vi "CreateExperimentRunsNode.vi"(8 "Error In":errorcluster, 10 "Experiment":T1={"File Path"=path "", "Operator"="Operator", "Project"="Project Description", "Target Dose (dpa)"=0.0, "Sample"={"Name"="", "Description"="", "Molar Mass (g/mol)"=0.0, "Density (g/cm^3)"=0.0, "Irradiation Area (cm^2)"=0.0, "SRIM Damage Peak (disp * ions/cm)"=0.0}, "Beam Line"={"Type"=enum."Ion Beam Analysis", "Ion"=enum."H", "Charge State"=0, "Total Source Ion Energy (kV)"=nan}, "Runs"=[]} {"Beam Line"."Charge State" min=1}, 11 "DOM Document In":refnum<k20>) -> (0 "Error out":errorcluster, 2 "Experiment Runs Node":refnum<k20>, 3 "DOM Document Out":refnum<k20>)   [LabVIEW 2012]
uses:
  Experiment.ctl
  Sample.ctl
  BeamLine.ctl
  BeamLineType.ctl
  BeamLineIon.ctl
  ExperimentRun.ctl
  ExperimentRunTiming.ctl
  ExperimentRunDose.ctl
  ExperimentRunFluence.ctl
  ExperimentRunTotalCharge.ctl
  <resource>/objmgr/DOMUserDefRef.rc
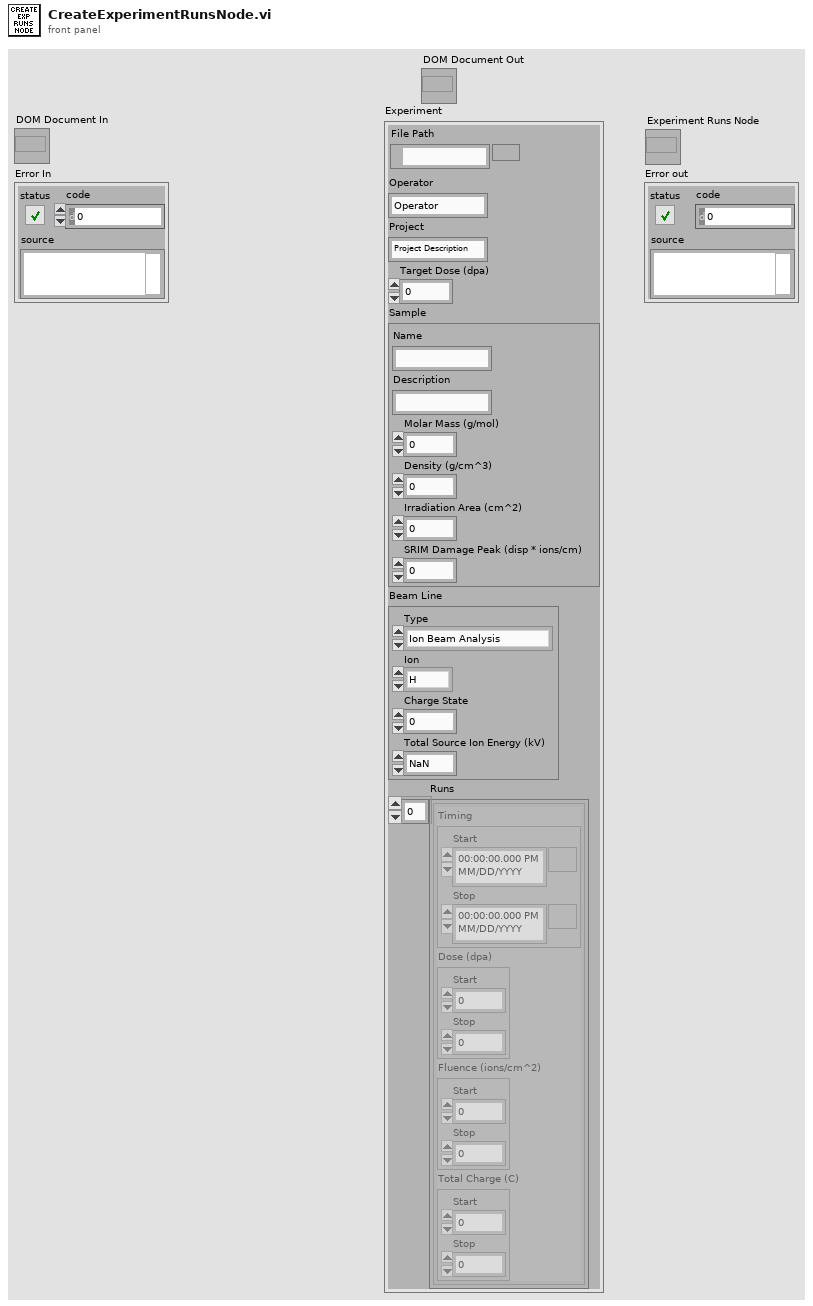
[diagram p1: front panel]
types:
  T1 = typedef "Experiment.ctl" = cluster{"File Path":path, "Operator":string, "Project":string, "Target Dose (dpa)":dbl, "Sample":T2, "Beam Line":T3, "Runs":T6[]}
  T2 = typedef "Sample.ctl" = cluster{"Name":string, "Description":string, "Molar Mass (g/mol)":dbl, "Density (g/cm^3)":dbl, "Irradiation Area (cm^2)":dbl, "SRIM Damage Peak (disp * ions/cm)":dbl}
  T3 = typedef "BeamLine.ctl" = cluster{"Type":T4, "Ion":T5, "Charge State":u8, "Total Source Ion Energy (kV)":dbl}
  T4 = typedef "BeamLineType.ctl" = enum16{"Ion Beam Analysis", "Auxiliary", "Radiation Damage"}
  T5 = typedef "BeamLineIon.ctl" = enum16{"H", "He", "C", "Fe", "Ni", "Pt", "Si", "Ag", "Au"}
  T6 = typedef "ExperimentRun.ctl" = cluster{"Timing":T7, "Dose (dpa)":T8, "Fluence (ions/cm^2)":T9, "Total Charge (C)":T10}
  T7 = typedef "ExperimentRunTiming.ctl" = cluster{"Start":timestamp, "Stop":timestamp}
  T8 = typedef "ExperimentRunDose.ctl" = cluster{"Start":dbl, "Stop":dbl}
  T9 = typedef "ExperimentRunFluence.ctl" = cluster{"Start":dbl, "Stop":dbl}
  T10 = typedef "ExperimentRunTotalCharge.ctl" = cluster{"Start":dbl, "Stop":dbl}
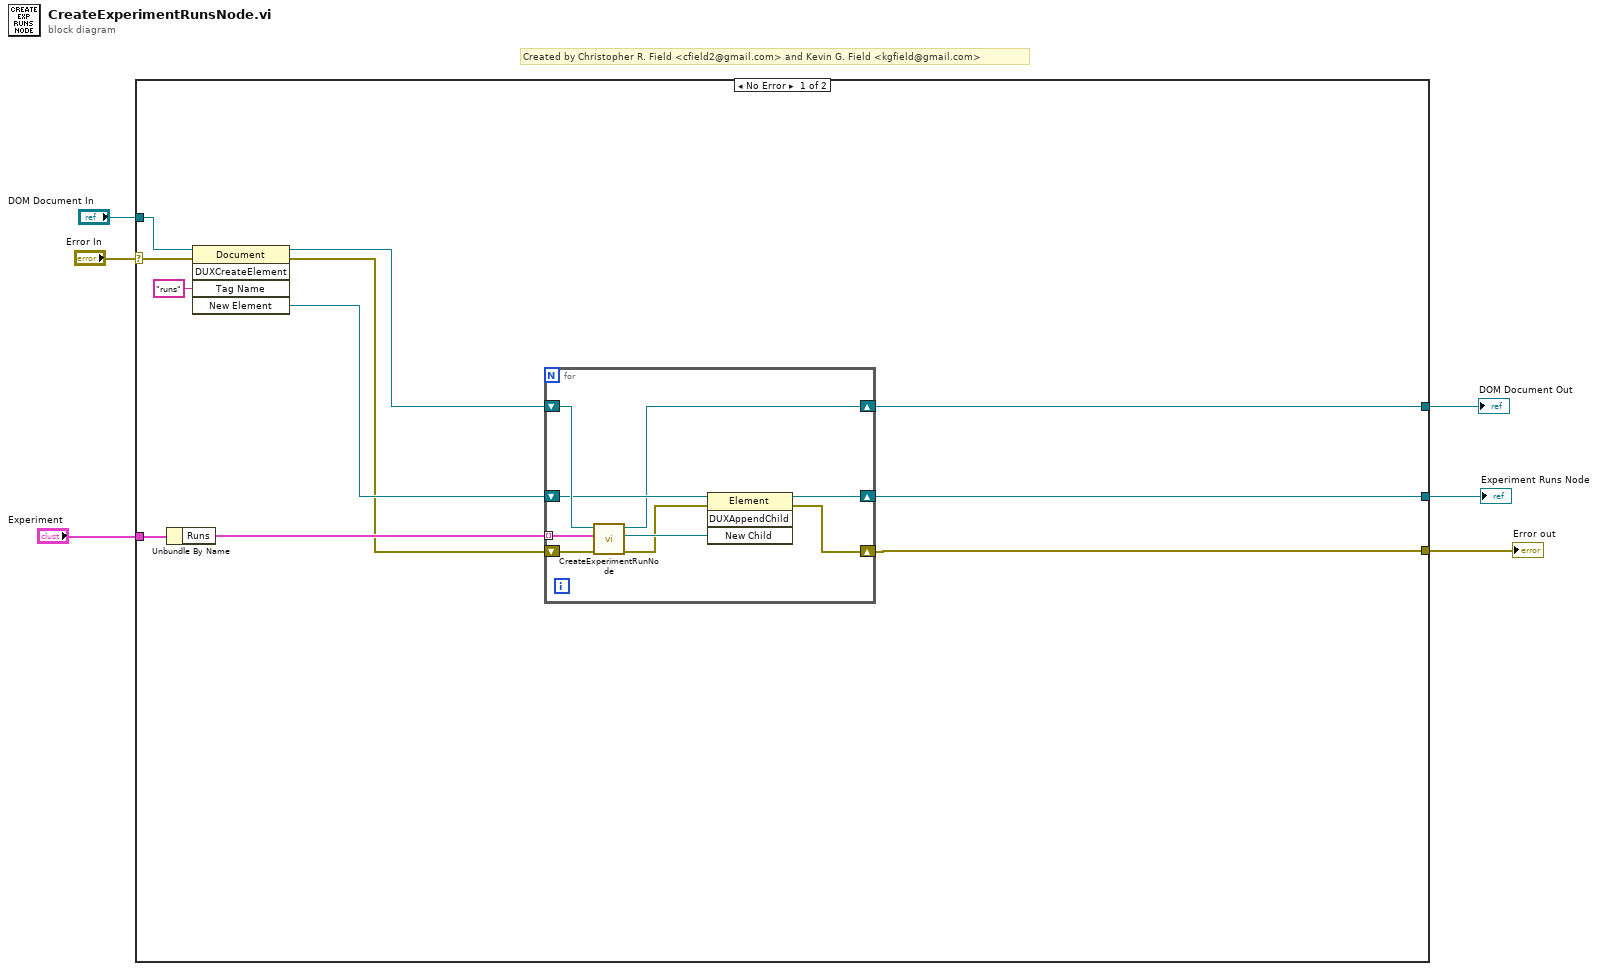
[diagram p0: block diagram]
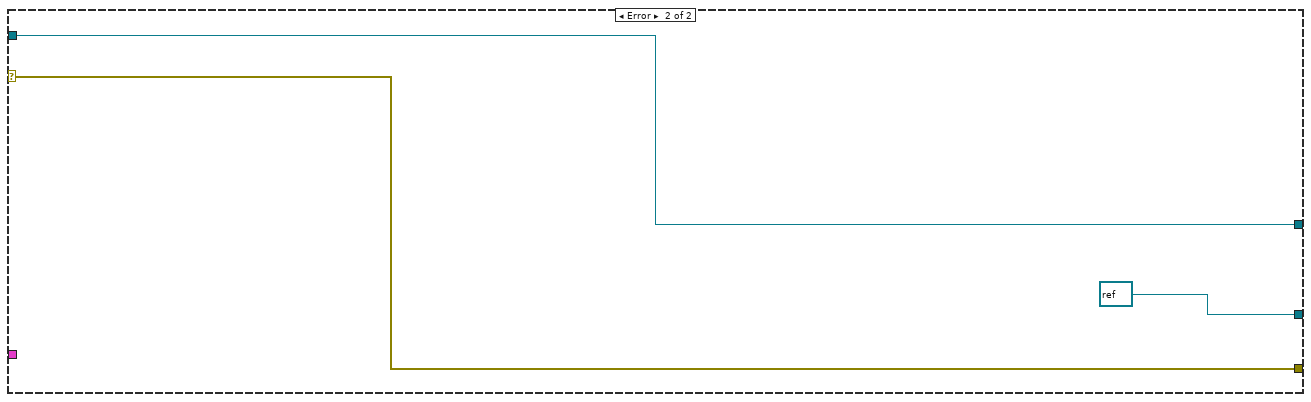
[diagram p2: hidden frame]
diagram:
  # "Created by Christopher R. Field <cfield2@gmail.com> and Kevin G. Field <kgfield@gmail.com>"
  n1 = case shown="No Error" "Error In" {
    selector: "Error In" -> [w15 w28]
    tunnel: "DOM Document In" -> [w17 w29]
    tunnel: [w8 refnum<k20> refnum ("Operator Node 2")] -> w5
    tunnel: [w9 w28] -> w4
    tunnel: [w7 w29] -> w2
    tunnel: "Experiment" -> [w14 _]
    frame No Error {
      n2 = Unbundle By Name(w14) -> ("Runs"=w13:T6[])
      n3 = invoke class="Document" method="DUXCreateElement"(reference=w17, error in=w15, "Tag Name"="runs") -> (reference out=w12:refnum<k20>, error out=w10:errorcluster, "New Element"=w11:refnum<k20>)  [unwired: 2 in, 2 out]
      n4 = for {
        tunnel: w13 -> [w26] mode=indexing
        shift-right: [w22] -> w7
        shift-left: w12 -> [w25]
        shift-right: [w21] -> w8
        shift-left: w11 -> [w23]
        shift-right: [w19] -> w9
        shift-left: w10 -> [w18]
        n5 = call "CreateExperimentRunNode.vi"("Error In"=w18, "Experiment Run"=w26, "DOM Document In"=w25) -> ("Error out"=w20:errorcluster, "Experiment Run Node"=w24:refnum<k20>, "DOM Document Out"=w22:refnum<k20>)  [unwired: 6 in]
        n6 = invoke class="Element" method="DUXAppendChild"(reference=w23, error in=w20, "New Child"=w24) -> (reference out=w21:refnum<k20>, error out=w19:errorcluster)  [unwired: 1 in, 2 out]
      }
    }
    frame Error {
    }
  }
  "Experiment Runs Node" <- w5
  "Error out" <- w4
  "DOM Document Out" <- w2
